vi "Build DIO Section from XML.vi"(4 "DIO Line Configs":u16[](array[numeric]), 6 "Channels":refnum<k24>[](array[refnum]), 8 "error in (no error)":errorcluster, 9 "Card Position in":T1 {"Slot #" max=15}, 10 "Name in":string, 11 "Node Ptr in":u64) -> (0 "error out":errorcluster)   [LabVIEW 2014, in "SLSC configuration System Explorer.lvlib"]
uses:
  SLSC configuration System Explorer.lvlib
  Type Defs/Card Position.ctl
  Shared/SPI Utility/Slot #.ctl
  C:/Files/Custom VeriStand Development/DET-SPI-Tool/XML Deserializer/SLSC Deserializer/SLSC Deserializer/bin/Release/SLSC Deserializer.dll
  XML Deserializer/SLSC Deserializer/SLSC Deserializer/bin/Release/SLSC Deserializer.dll
  <vilib>/NI Veristand/Custom Device API/Custom Device Channel.ctl
  <vilib>/NI Veristand/Custom Device API/Custom Device Channel Type.ctl
  Shared/Constants.vi
  <vilib>/NI Veristand/Custom Device API/Set Item Property (U16).vi
  <vilib>/NI Veristand/Custom Device API/Custom Device API.lvlib
  Shared/SLSC configuration Shared.lvlib
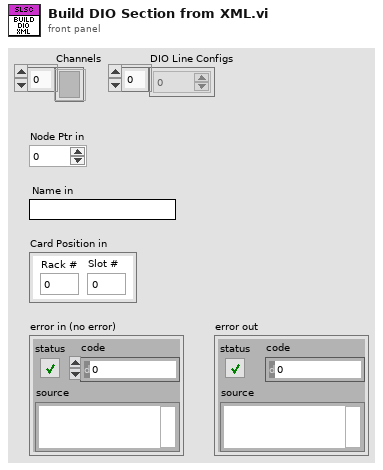
[diagram p1: front panel]
types:
  T1 = typedef "SLSC configuration Shared.lvlib/Card Position.ctl" = cluster{"Rack #":u8, "Slot #":T2}
  T2 = typedef "SLSC configuration Shared.lvlib/Slot #.ctl" = u8
  T3 = typedef "Custom Device API.lvlib/Custom Device Channel Type.ctl" = enum16{"Input", "Output"}
  T4 = typedef "Custom Device API.lvlib/Custom Device Channel.ctl" = cluster{"Type":T3, "Units":string, "Default Value":dbl, "Faultable":bool, "Scalable":bool}
  T5 = typedef "Custom Device API.lvlib/Custom Device Item Ref.ctl" = u64
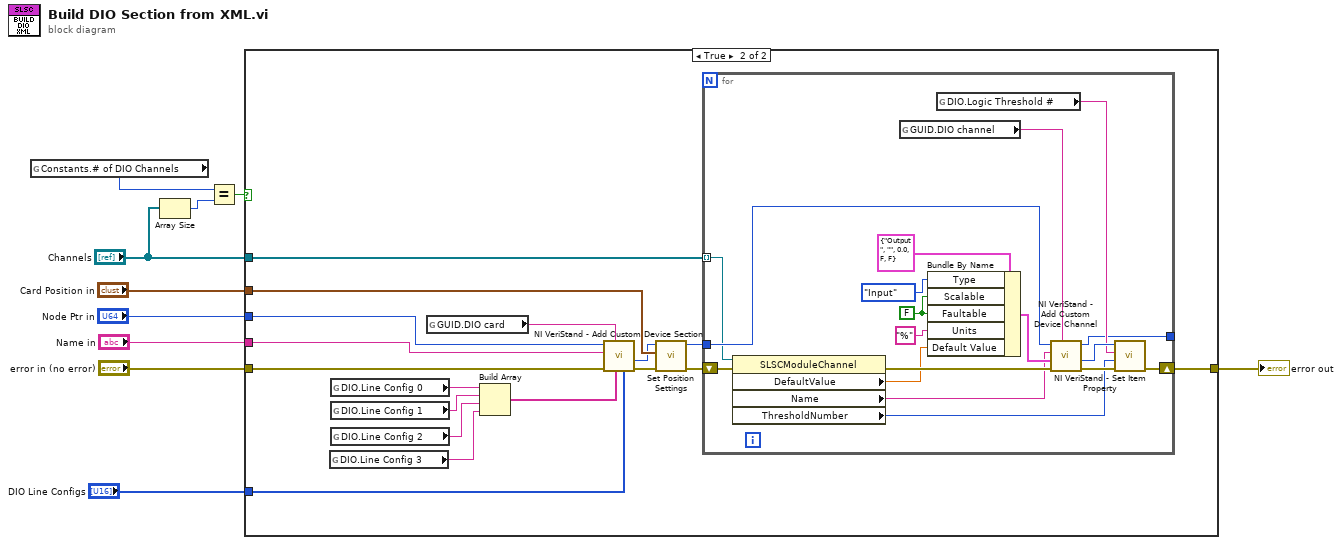
[diagram p0: block diagram]
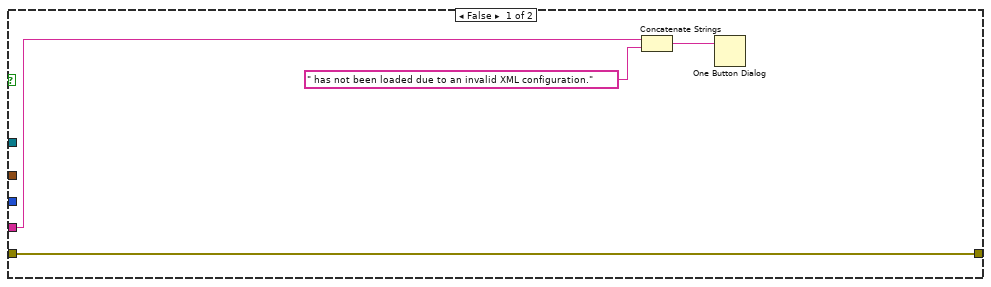
[diagram p2: hidden frame]
diagram:
  n1 = global read "Constants.vi" "Constants.# of DIO Channels"() -> (w3:u8)
  n2 = Array Size(array="Channels") -> (size(s)=w4:i32)
  n3 = Equal?(x=w3, y=w4) -> (x = y?=w2:bool)
  n4 = case shown="True" w2 {
    tunnel: "Card Position in" -> [_ w31]
    tunnel: "Node Ptr in" -> [_ w30]
    tunnel: "Name in" -> [w12 w29]
    tunnel: "error in (no error)" -> [w11 w28]
    tunnel: "Channels" -> [_ w17]
    tunnel: "DIO Line Configs" -> [_ w16]
    tunnel: [w11 w15] -> w5
    frame False {
      n5 = Concatenate Strings(w12, " has not been loaded due to an invalid XML configuration." ("string")) -> (w13:string)
      n6 = One Button Dialog(message=w13) -> ()  [unwired: 1 in, 1 out]
    }
    frame True {
      n7 = global read "Constants.vi" "DIO.Line Config 3"() -> (w19:string)
      n8 = global read "Constants.vi" "DIO.Line Config 0"() -> (w22:string)
      n9 = global read "Constants.vi" "DIO.Line Config 1"() -> (w21:string)
      n10 = global read "Constants.vi" "DIO.Line Config 2"() -> (w20:string)
      n11 = global read "Constants.vi" "GUID.DIO card"() -> (w27:string)
      n12 = Build Array(w22, w21, w20, w19) -> (w18:string[])
      n13 = call <vilib>:"NI VeriStand - Add Custom Device Section.vi"("Property Values"=w16, "Property names"=w18, "GUID (Default Section)"=w27, "error in (no error)"=w28, "Section Name"=w29, "Parent Ref in"=w30) -> ("error out"=w26:errorcluster, "Section Ptr"=w25:T5)  [unwired: 2 in, 2 out]
      n14 = call "Set Position Settings.vi"("error in (no error)"=w26, "Card Position"=w31, "Item Ref in"=w25) -> ("error out"=w23:errorcluster, "Item Ref out"=w24:T5)  [unwired: 7 in]
      n15 = for {
        shift-right: [w46] -> w15
        shift-left: w23 -> [w36]
        tunnel: w24 -> [w49]
        tunnel: [w39] -> _
        tunnel: w17 -> [w37] mode=indexing
        w40 = FALSE ("Scalable")
        n16 = property class="SLSCModuleChannel"(reference=w37, error in=w36) -> (error out=w35:errorcluster, "DefaultValue"=w32:dbl, "Name"=w33:string, "ThresholdNumber"=w34:u8)  [unwired: 1 out]
        n17 = global read "Constants.vi" "GUID.DIO channel"() -> (w48:string)
        n18 = Bundle By Name(cluster=T4 {"Type"=enum."Output", "Units"="", "Default Value"=0.0, "Faultable"=FALSE, "Scalable"=FALSE} ("Channel"), "Type"=Custom_Device_Channel_Type."Input", "Scalable"=w40, "Faultable"=w40, "Units"="%", "Default Value"=w32) -> (w42:T4)
        n19 = global read "Constants.vi" "DIO.Logic Threshold #"() -> (w44:string)
        n20 = call <vilib>:"NI VeriStand - Add Custom Device Channel.vi"("GUID (Default Channel)"=w48, "error in (no error)"=w35, "Channel"=w42, "Channel Name"=w33, "Parent Ref in"=w49) -> ("error out"=w47:errorcluster, "Channel Ref"=w45:T5, "Parent Ref out"=w39:T5)  [unwired: 3 in, 1 out]
        n21 = call-poly <vilib>:"NI VeriStand - Set Item Property.vi"("error in (no error)"=w47, "Value"=w34, "Property Name"=w44, "Item Ref in"=w45) -> ("error out"=w46:errorcluster)  [unwired: 5 in, 2 out]
      }
    }
  }
  "error out" <- w5
